vi "Stop Control v3.vi"(9 "Rate (unit/s)":dbl=0.2, 10 "Loop Time (ms)":u32=10, 11 "Recieved Motor Input":dbl) -> (2 "Done Stopping":bool, 3 "New Motor Input":dbl)   [LabVIEW 2011]
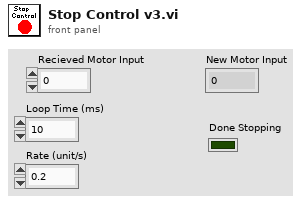
[diagram p1: front panel]
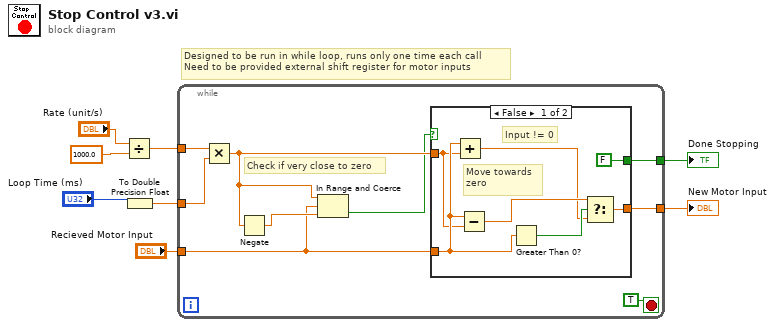
[diagram p0: block diagram]
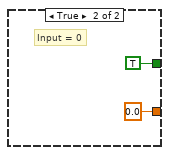
[diagram p2: hidden frame]
diagram:
  # "Designed to be run in while loop, runs only one time each call\nNeed to be provided external shift register for motor inputs"
  n1 = Divide(x="Rate (unit/s)", y=1000.0) -> (x/y=w4:dbl)
  n2 = To Double Precision Float(number="Loop Time (ms)") -> (double precision float=w1:dbl)
  n3 = while {
    tunnel: w4 -> [w14]
    tunnel: [w17] -> w8
    tunnel: [w16] -> w7
    tunnel: w1 -> [w13]
    tunnel: "Recieved Motor Input" -> [w10]
    stop <- TRUE stop-if-true
    # "Check if very close to zero"
    n4 = Multiply(x=w14, y=w13) -> (x*y=w11:dbl)
    n5 = Negate(x=w11) -> (-x=w12:dbl)
    n6 = In Range and Coerce(upper limit=w11, x=w10, lower limit=w12) -> (In Range?=w9:bool)  [unwired: 1 out]
    n7 = case shown="False" w9 {
      tunnel: [w18 0.0] -> w16
      tunnel: w11 -> [w20 _]
      tunnel: w10 -> [w21 _]
      tunnel: [FALSE TRUE] -> w17
      frame False {
        # "Move towards\nzero"
        # "Input != 0"
        n8 = Add(x=w21, y=w20) -> (x+y=w19:dbl)
        n9 = Subtract(x=w21, y=w20) -> (x-y=w22:dbl)
        n10 = Greater Than 0?(x=w21) -> (x > 0?=w23:bool)
        n11 = Select(t=w22, s=w23, f=w19) -> (s? t:f=w18:dbl)
      }
      frame True {
        # "Input = 0"
      }
    }
  }
  "Done Stopping" <- w8
  "New Motor Input" <- w7
